vi "Sequence.GetiStepProperties.vi"(7 "Iteration":string, 8 "error in (no error)":errorcluster, 11 "Elements":T1[](array[typedef])) -> (0 "error out":errorcluster, 1 "Step Conatins iStep?":bool, 3 "iStepForLoop Ref":refnum<k24>)   [LabVIEW 2013, in "Simple Sequence Tools - Editor.lvlib"]
uses:
  Simple Sequence Tools - Editor.lvlib
  Types/Compiled.StepElementProperties.ctl
  Shared/Types/ChannelProperties.ctl
  Shared/Types/StepTypes.ctl
  NationalInstruments.VeriStand.RealTimeSequenceDefinitionApi
  <vilib>/Analysis/1siggen.llb/Ramp Pattern by Delta.vi
  Shared/SubVIs/Constants.vi
  Shared/Simple Sequence Tools - Shared.lvlib
  <vilib>/Analysis/NI_AALBase.lvlib
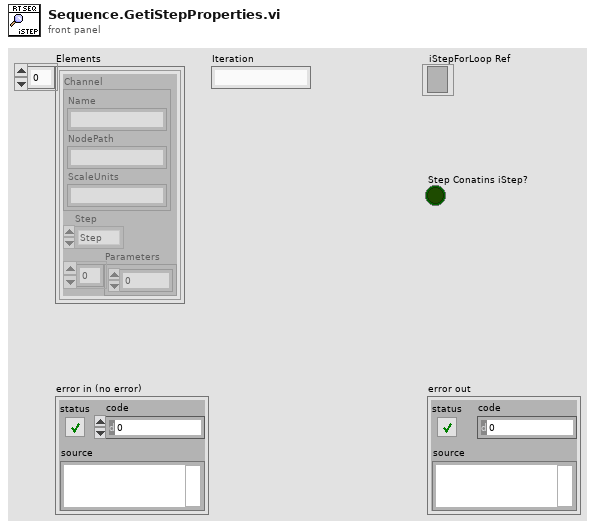
[diagram p1: front panel]
types:
  T1 = typedef "Simple Sequence Tools - Editor.lvlib/Compiled.StepElementProperties.ctl" = cluster{"Channel":T2, "Step":T3, "Parameters":dbl[]}
  T2 = typedef "Simple Sequence Tools - Shared.lvlib/ChannelProperties.ctl" = cluster{"Name":string, "NodePath":string, "ScaleUnits":string}
  T3 = typedef "Simple Sequence Tools - Shared.lvlib/StepTypes.ctl" = enum8{"Step", "iStep", "Ramp", "Unchanged", "Unknown"}
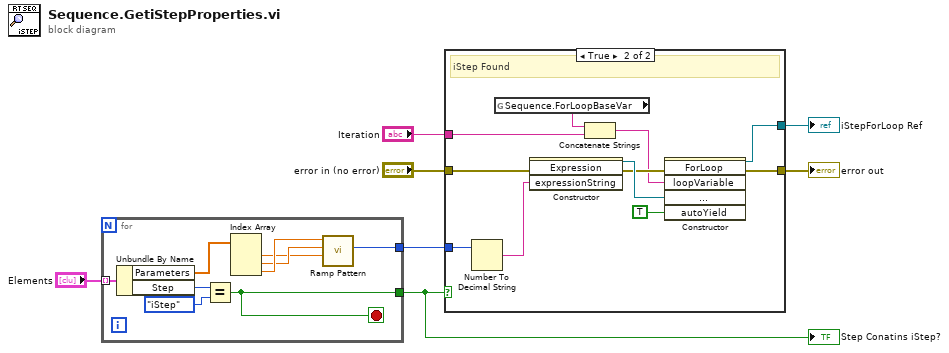
[diagram p0: block diagram]
diagram:
  n1 = for {
    tunnel: "Elements" -> [w16] mode=indexing
    tunnel: [w9] -> w5
    tunnel: [w8] -> w3
    stop <- w8 stop-if-true
    n2 = Unbundle By Name(w16) -> ("Parameters"=w10:dbl[], "Step"=w15:T3)
    n3 = Equal?(x=w15, y=StepTypes."iStep") -> (x = y?=w8:bool)
    n4 = Index Array(array=w10) -> (element #1=w11:dbl, element #2=w12:dbl, element #3=w13:dbl)  [unwired: 3 in]
    n5 = call-poly <vilib>:"Ramp Pattern.vi"("start"=w11, "end"=w12, "delta"=w13) -> ("samples"=w9:i32)  [unwired: 6 in, 2 out]
  }
  "Step Conatins iStep?" <- w3
  n6 = case shown="True" w3 {
    tunnel: "error in (no error)" -> [w17 w26]
    tunnel: [w17 w25] -> w6
    tunnel: w5 -> [_ w24]
    tunnel: [_ w22] -> w4
    tunnel: "Iteration" -> [_ w20]
    frame False {
      # "No iStep in step"
    }
    frame True {
      # "iStep Found"
      n7 = Number To Decimal String(number=w24) -> (decimal integer string=w23:string)  [unwired: 1 in]
      n8 = global read "Constants.vi" "Sequence.ForLoopBaseVar"() -> (w18:string)
      n9 = constructor class="Expression"(error in=w26, "expressionString"=w23) -> (reference out=w28:refnum<k24>, error out=w27:errorcluster)  [unwired: 2 in, 2 out]
      n10 = Concatenate Strings(w18, w20) -> (w19:string)
      n11 = constructor class="ForLoop"(error in=w27, "loopVariable"=w19, "iterations"=w28, "autoYield"=TRUE) -> (reference out=w22:refnum<k24>, error out=w25:errorcluster)  [unwired: 2 in, 4 out]
    }
  }
  "error out" <- w6
  "iStepForLoop Ref" <- w4
